vi "HTTP_SetAuthorizationHeader.vi"(0 "client handle":T1, 7 "JWT":string, 11 "error in (no error)":errorcluster) -> (4 "client handle dup":T1, 15 "error out":errorcluster)   [LabVIEW 2017, in "JSONWebToken.lvclass"]
uses:
  JSONWebToken.lvclass
  <vilib>/httpClient/ClientHandle.ctl
  <vilib>/httpClient/LabVIEWHTTPClient.lvlib
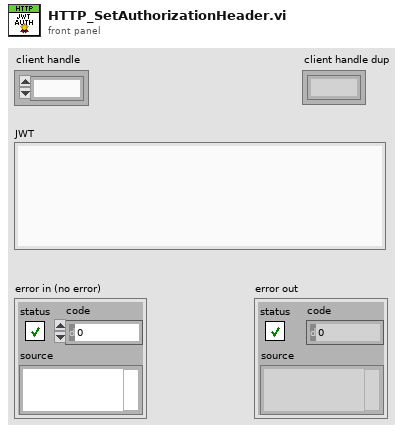
[diagram p1: front panel]
types:
  T1 = typedef "LabVIEWHTTPClient.lvlib/ClientHandle.ctl" = refnum<k1>
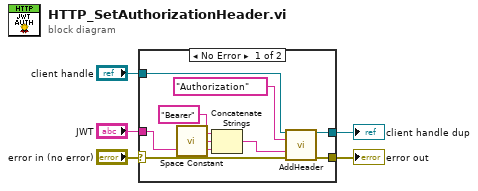
[diagram p0: block diagram]
diagram:
  n1 = case shown="No Error" "error in (no error)" {
    selector: "error in (no error)" -> [w7 w16]
    tunnel: [w6 w16] -> w3
    tunnel: [w9 w15] -> w4
    tunnel: "client handle" -> [w10 w15]
    tunnel: "JWT" -> [w8 _]
    frame No Error {
      n2 = call <vilib>:"Space Constant.vi"() -> ("String"=w13:string)
      n3 = Concatenate Strings("Bearer" ("path"), w13, w8) -> (w11:string)
      n4 = call <vilib>:"AddHeader.vi"("client handle"=w10, "header"="Authorization", "value"=w11, "error in (no error)"=w7) -> ("client handle out"=w9:T1, "error out"=w6:errorcluster)  [unwired: 10 in]
    }
    frame Error {
    }
  }
  "error out" <- w3
  "client handle dup" <- w4
